vi "Variant To Key Info.vi"(4 "Registry Variant Accessor in":refnum<class "CConfig Variant Accessor.lvclass">, 6 "Variant":variant, 8 "error in (no error)":errorcluster, 11 "Carya Config in":refnum<class "Carya Config.lvclass">) -> (0 "error out":errorcluster, 1 "Keys":string[](array[string]), 2 "Sections":string[](array[string]), 3 "Carya Config out":refnum<class "Carya Config.lvclass">, 5 "Valid Label?":bool[](array[boolean]), 7 "Found?":bool[](array[boolean]))   [LabVIEW 2013, in "Carya Config.lvclass"]
doc: "Copyright 2018, Carya Automatisering, Wiebe Walstra."
uses:
  Carya Config.lvclass
  CConfig Variant Accessor/CConfig Variant Accessor.lvclass
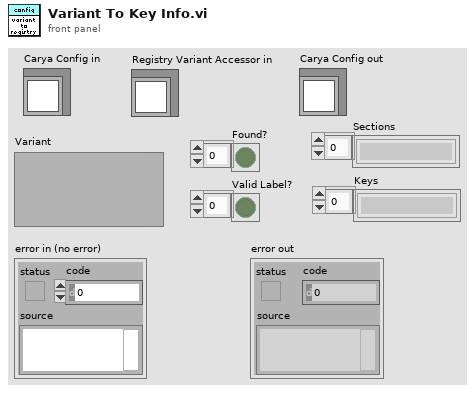
[diagram p1: front panel]
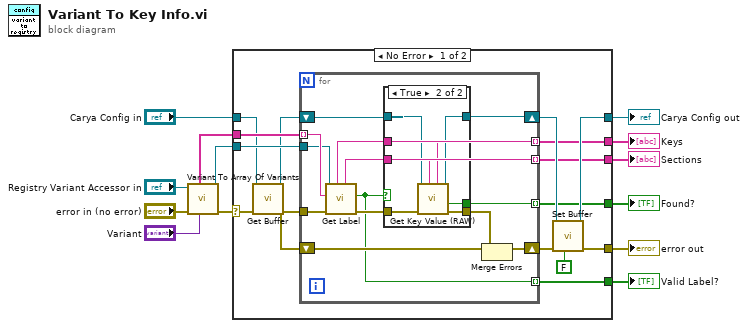
[diagram p0: block diagram]
diagram:
  n1 = call-dynamic "Variant To Array Of Variants.vi"("Variant"="Variant", "error in (no error)"="error in (no error)", "Registry Variant Accessor in"="Registry Variant Accessor in") -> ("error out"=w5:errorcluster, "Registry Variant Accessor out"=w9:refnum<class "CConfig Variant Accessor.lvclass">, "Labels (RAW)"=w10:string[])  [unwired: 3 in, 3 out]
  n2 = case shown="No Error" w5 {
    selector: w5 -> [w21 w52]
    tunnel: w10 -> [w28 _]
    tunnel: w9 -> [w27 _]
    tunnel: "Carya Config in" -> [w24 w51]
    tunnel: [w23 w52] -> w7
    tunnel: [w22 w51] -> w6
    tunnel: [w17 _] -> w4
    tunnel: [w16 _] -> w3
    tunnel: [w15 _] -> w2
    tunnel: [w14 _] -> w1
    frame No Error {
      n3 = call-dynamic "Get Buffer.vi"("error in (no error)"=w21, "Carya Config in"=w24) -> ("error out"=w25:errorcluster, "Config"=w20:refnum<class "Carya Config.lvclass">)  [unwired: 8 in]
      n4 = for {
        tunnel: [w29] -> w15 mode=indexing
        tunnel: [w37] -> w14 mode=indexing
        tunnel: w25 -> [w41]
        tunnel: w28 -> [w40] mode=indexing
        tunnel: w27 -> [w39]
        tunnel: [w31] -> w16 mode=indexing
        tunnel: [w30] -> w17 mode=indexing
        shift-right: [w34] -> w26
        shift-left: w25 -> [w36]
        shift-right: [w32] -> w19
        shift-left: w20 -> [w33]
        n5 = call-dynamic "Get Label.vi"("error in (no error)"=w41, "Label"=w40, "Registry Variant Accessor in"=w39) -> ("error out"=w38:errorcluster, "Valid?"=w29:bool, "Section out"=w31:string, "Key out"=w30:string)  [unwired: 3 in, 2 out]
        n6 = case shown="True" w29 {
          tunnel: [w42 w44] -> w35
          tunnel: [w43 w46] -> w32
          tunnel: w38 -> [w42 w49]
          tunnel: w31 -> [_ w48]
          tunnel: w30 -> [_ w47]
          tunnel: w33 -> [w43 w50]
          tunnel: [_ w45] -> w37
          frame False {
          }
          frame True {
            n7 = call-dynamic "Get Key Value (RAW).vi"("Key name"=w47, "Section name"=w48, "error in (no error)"=w49, "Carya Config in"=w50) -> ("error out"=w44:errorcluster, "Found?"=w45:bool, "Carya Config out"=w46:refnum<class "Carya Config.lvclass">)  [unwired: 4 in, 1 out]
          }
        }
        n8 = Merge Errors(w36, w35) -> (w34:errorcluster)
      }
      n9 = call-dynamic "Set Buffer.vi"("Set? [T]"=FALSE, "error in (no error)"=w26, "Carya Config"=w19) -> ("error out"=w23:errorcluster, "Carya Config out"=w22:refnum<class "Carya Config.lvclass">)  [unwired: 7 in]
    }
    frame Error {
    }
  }
  "error out" <- w7
  "Carya Config out" <- w6
  "Found?" <- w1
  "Valid Label?" <- w2
  "Sections" <- w3
  "Keys" <- w4
